vi "Elevator Motion Profile.vi"   [LabVIEW 2017]
uses:
  Robot Global Data.vi
  <vilib>/Rock Robotics/WPI/ThirdParty/Phoenix-LabVIEW/Motor Controller/Get/CTRE_Phoenix_MotorController_GetGeneralStatus.vi
types:
  T1 = typedef "Dashboard Control Data.ctl" = cluster{"Drivetrain Settings Cluster":T2, "Intake Presets":T5, "Elevator Settings Cluster":T6, "Drivetrain Encoder Values":T8, "Auton Chooser":T9, "Auton Presets":cluster{"Start Position":dbl}, "Elevator Encoder Values":T10, "Pressure M":dbl, "Pressure B":dbl, "Zero All?":bool, "Enable Vision":bool}
  T2 = typedef "Drivetrain Settings Cluster.ctl" = cluster{"Gyro Steer PID Gains":T3, "Distance Drive PID Gains":T3, "Drive Tolerance":dbl, "Gyro Tolerance":dbl, "Gyro Output":dbl, "Distance Output":dbl, "Y Power Multiplier":dbl, "Turn Power Multiplier":dbl, "Creep Rate":dbl, "Encoder Reset":bool, "DT Mode Modifier":enum16{"None, Default", "Cube", "Square"}, "Left Encoder Tick Constant":dbl, "Right Encoder Tick Constant":dbl, "Shift Speed":dbl, "Zero Gyro":bool, "Y min":dbl, "Y max":dbl, "X min":dbl, "X max":dbl, "Finish Velocity":dbl, "Anti-Tip Settings":T4}
  T3 = typedef "PID Gains Cluster.ctl" = cluster{"Proportional Gain":dbl, "Integral Time":dbl, "Derivative Time":dbl}
  T4 = typedef "Anti-Tip Settings.ctl" = cluster{"Pitch Tip Constant":dbl, "Wheel Diameter":dbl, "Gearbox Reduction":dbl, "Motor Count":dbl, "Mass of Robot":dbl, "Almost Tip Constant":dbl, "Dist to CG":dbl}
  T5 = typedef "Intake Presets.ctl" = cluster{"Idle Angle":dbl, "Mid Angle":dbl, "Low Angle":dbl, "Outtake Power":dbl, "Intake Power":dbl, "Unstuck":dbl, "Angle Tolerance":dbl, "Max Angle":dbl, "Max Current":dbl, "Current Trip Time":dbl, "Reset Encoder?":bool, "Encoder Scale":dbl, "PID gains":cluster{"proportional gain (Kc)":dbl, "integral time (Ti, min)":dbl, "derivative time (Td, min)":dbl}, "output range":cluster{"output high":dbl, "output low":dbl}, "IR Constant Pull Rate":dbl, "Shoot Angle":dbl, "Shoot High":dbl, "Manual Limit":dbl}
  T6 = typedef "Elevator Settings Cluster.ctl" = cluster{"Ground Height":dbl, "Switch Height":dbl, "Scale High Height ":dbl, "Scale Low Height":dbl, "Elevator PID Gains":T7, "Elevator Tolerance":dbl, "Reset Encoders":bool, "Encoder Scale":dbl, "Max Height":dbl, "Mid Height":dbl, "output range":cluster{"output high":dbl, "output low":dbl}, "Upper Slow Down Tolerance":dbl, "Tick Constant":dbl, "Tip Constant":dbl, "Slow Down Multiplier":dbl, "Almost Tip Constant":dbl, "Bottom Trip Offset":dbl, "Lower Slow Down Tolerance":dbl, "Cruise Velocity":dbl, "Max Acceleration":dbl, "Feed Forward":dbl}
  T7 = typedef "PID Gains.ctl" = cluster{"proportional gain (Kc)":dbl, "integral time (Ti, min)":dbl, "derivative time (Td, min)":dbl}
  T8 = typedef "DT Encoder Values.ctl" = cluster{"Left Encoder":cluster{"Distance":dbl, "Speed":dbl, "Tick":dbl}, "Right Encoder":cluster{"Distance":dbl, "Speed":dbl, "Tick":dbl}}
  T9 = typedef "Auton Chooser.ctl" = cluster{"Left":bool, "Center":bool, "Right":bool, "Scale":bool, "Both":bool, "Switch":bool, "Test":bool, "No Script":bool, "Drive PID":bool, "Elevator PID":bool, "Gyro PID":bool, "Drive Forward":bool, "Switch Cross Front":bool}
  T10 = typedef "Elevator Encoder Values.ctl" = cluster{"Encoder Values":cluster{"Distance":dbl, "Speed":dbl, "Tick":dbl}}
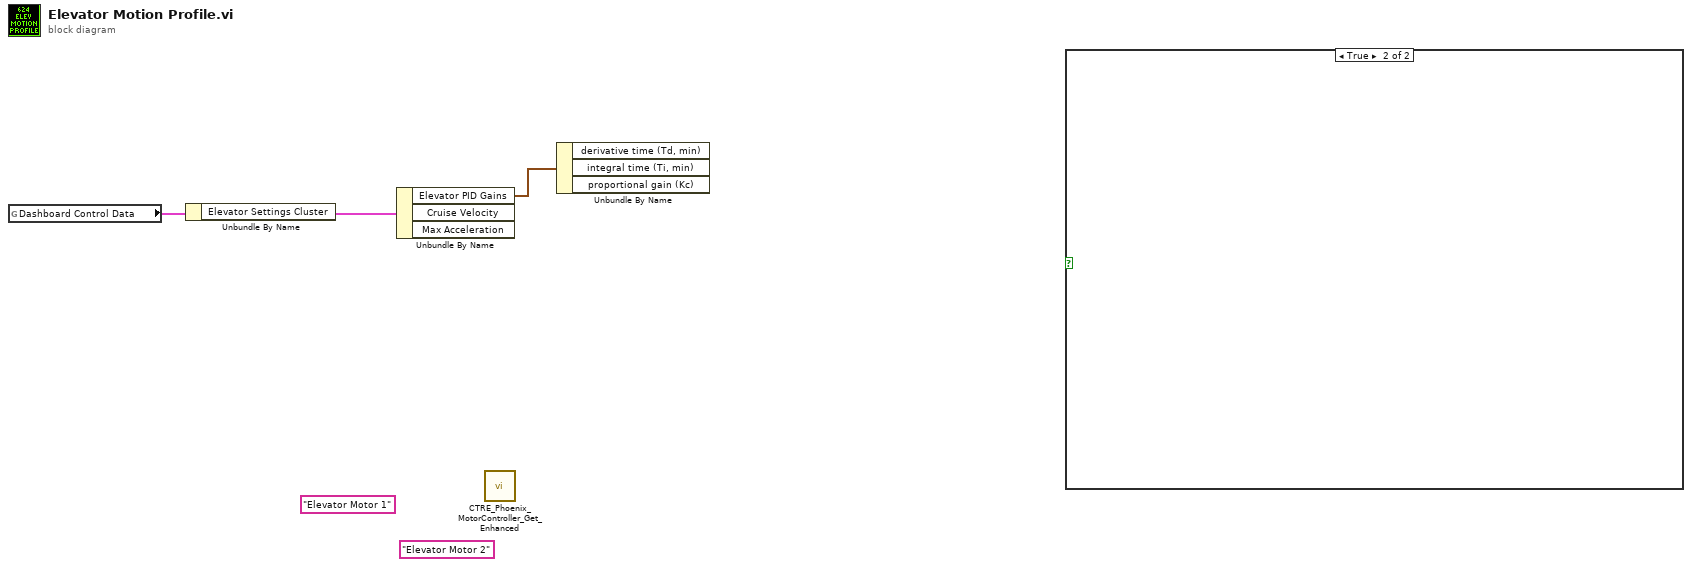
[diagram p0: block diagram]
diagram:
  (unwired) "Elevator Motor 2" ("refnum name")
  (unwired) "Elevator Motor 1" ("refnum name")
  n1 = global read "Robot Global Data.vi" "Dashboard Control Data"() -> (w3:T1)
  n2 = Unbundle By Name(w3) -> ("Elevator Settings Cluster"=w2:T6)
  n3 = Unbundle By Name(w2) -> ("Elevator PID Gains"=w1:T7)  [unwired: 2 out]
  n4 = call-poly <vilib>:"CTRE_Phoenix_MotorController_Get_Enhanced.vi"() -> ()  [unwired: 10 in, 6 out]
  n5 = Unbundle By Name(w1) -> ()  [unwired: 3 out]
  n6 = case shown="True" {
    selector: _ -> [_ _]
    frame False {
    }
    frame True {
    }
  }
